vi "RT-Cut-String.vi"(2 "Input string":string="﻿<?xml version=\"1.0\" encoding=\"utf-8\"?>\n<root>\n  <item>\n    <title>input_layer.weight</title>\n    <data>-0.035094768,-0.042544693,-0.015341377,-0.04649648</data>\n  </item>\n  <item>\n    <title>input_layer.bias</title>\n    <data>-0.01824686,-0.023881253,-0.045103975,0.01384796</data>\n  </item>\n  <item>\n    <title>lstm1.weight_ih_l0</title>\n    <data>-0.03255939,-0.16730139,0.0048500034,-0.21278836</data>\n  </item>\n  <item>\n    <title>lstm1.weight_hh_l0</title>\n    <data>0.23438185,0.18135086,-0.19734596,0.0075714383</data>\n  </item>\n  <item>\n    <title>lstm1.bias_ih_l0</title>\n    <data>0.11472153,0.05598353,0.17399026,0.07533772,0.078231476</data>\n  </item>\n  <item>\n    <title>lstm1.bias_hh_l0</title>\n    <data>-0.049843445,0.12087957,-0.106307246,0.21267405,0.21193506</data>\n  </item>\n  <item>\n    <title>lstm2.weight_ih_l0</title>\n    <data>0.3794311,-1.5752678,0.13325751,1.6159518,-0.27572358,0.2268258,0.3473175</data>\n  </item>\n  <item>\n    <title>lstm2.weight_hh_l0</title>\n    <data>0.10963432,-0.2202571,0.1343695,-0.18129872,-0.0493728</data>\n  </item>\n  <item>\n    <title>lstm2.bias_ih_l0</title>\n    <data>-1.7883135,-2.044432,-1.7003092,-1.6104138,-2.149785</data>\n  </item>\n  <item>\n    <title>lstm2.bias_hh_l0</title>\n    <data>-1.6704968,-2.138146,-1.6832165,-1.9645302,-1.8487101,-2.2139163,-1.9057949</data>\n  </item>\n  <item>\n    <title>output_layer.weight</title>\n    <data>0.33229554,-0.40919906,-0.010906305,-0.48219386,0.22490042,0.2636983</data>\n  </item>\n  <item>\n    <title>output_layer.bias</title>\n    <data>-0.33105168,-0.34130678,-0.39349645,-0.4524786</data>\n  </item>\n</root>", 3 "End Cut":string="</data>", 4 "Start Cut":string="<data>") -> (0 "Remainder":string, 1 "Extracted":string)   [LabVIEW 2020]
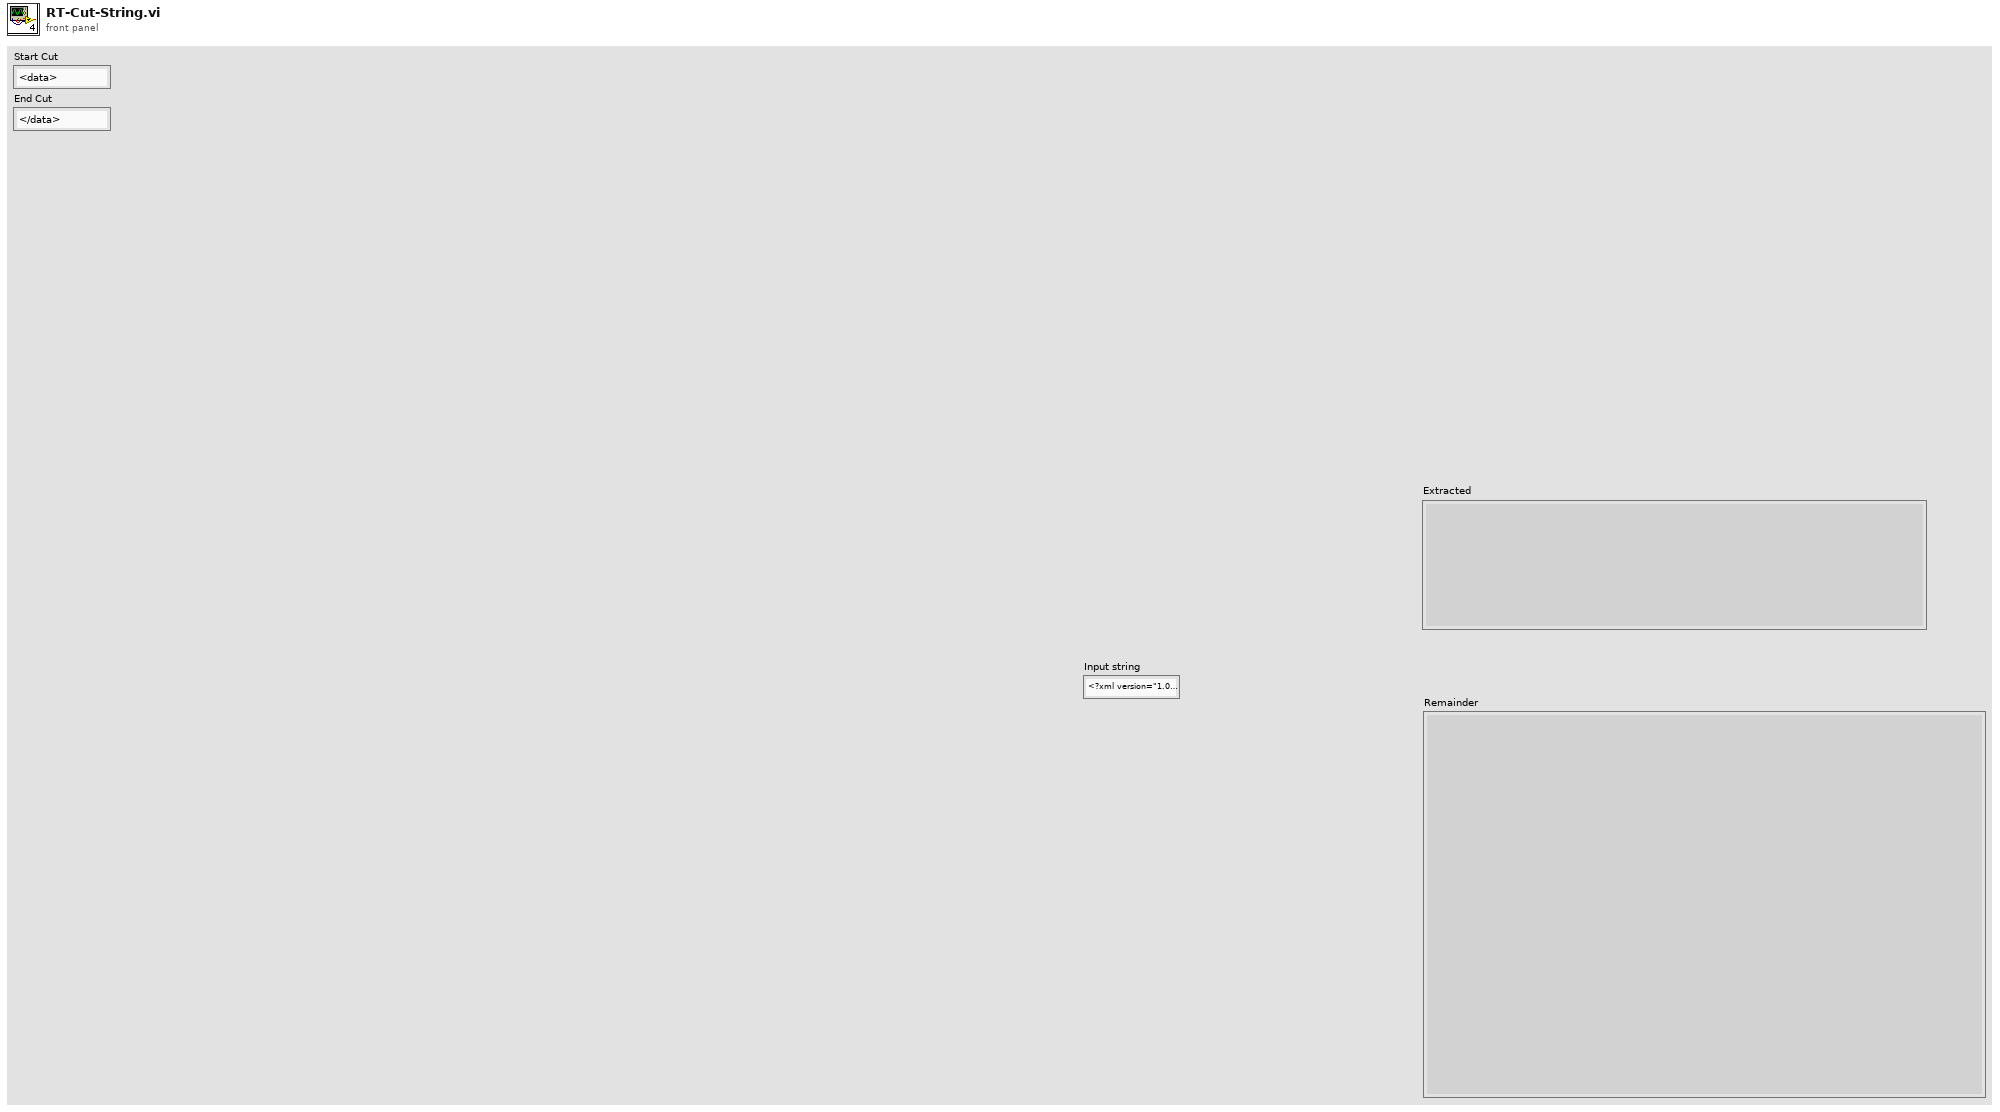
[diagram p1: front panel]
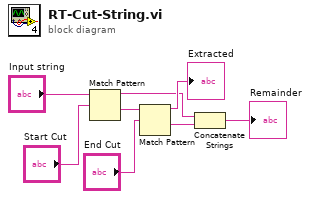
[diagram p0: block diagram]
diagram:
  n1 = Match Pattern(string="Input string", regular expression="Start Cut") -> (before substring=w1:string, after substring=w6:string)  [unwired: 1 in, 2 out]
  n2 = Match Pattern(string=w6, regular expression="End Cut") -> (before substring=→"Extracted":string, after substring=w2:string)  [unwired: 1 in, 2 out]
  n3 = Concatenate Strings(w1, w2) -> (→"Remainder":string)
